vi "Auto Reziseable UI.vi"() -> ()   [LabVIEW 2010]
uses:
  <vilib>/Utility/miscctls.llb/LVPointTypeDef.ctl
  <vilib>/Utility/miscctls.llb/LVRectTypeDef.ctl
panel:
  out "Waveform Graph":i32[](graph)
  out "Front Panel Window:Window Bounds":T1
  in  "Stop Button":bool
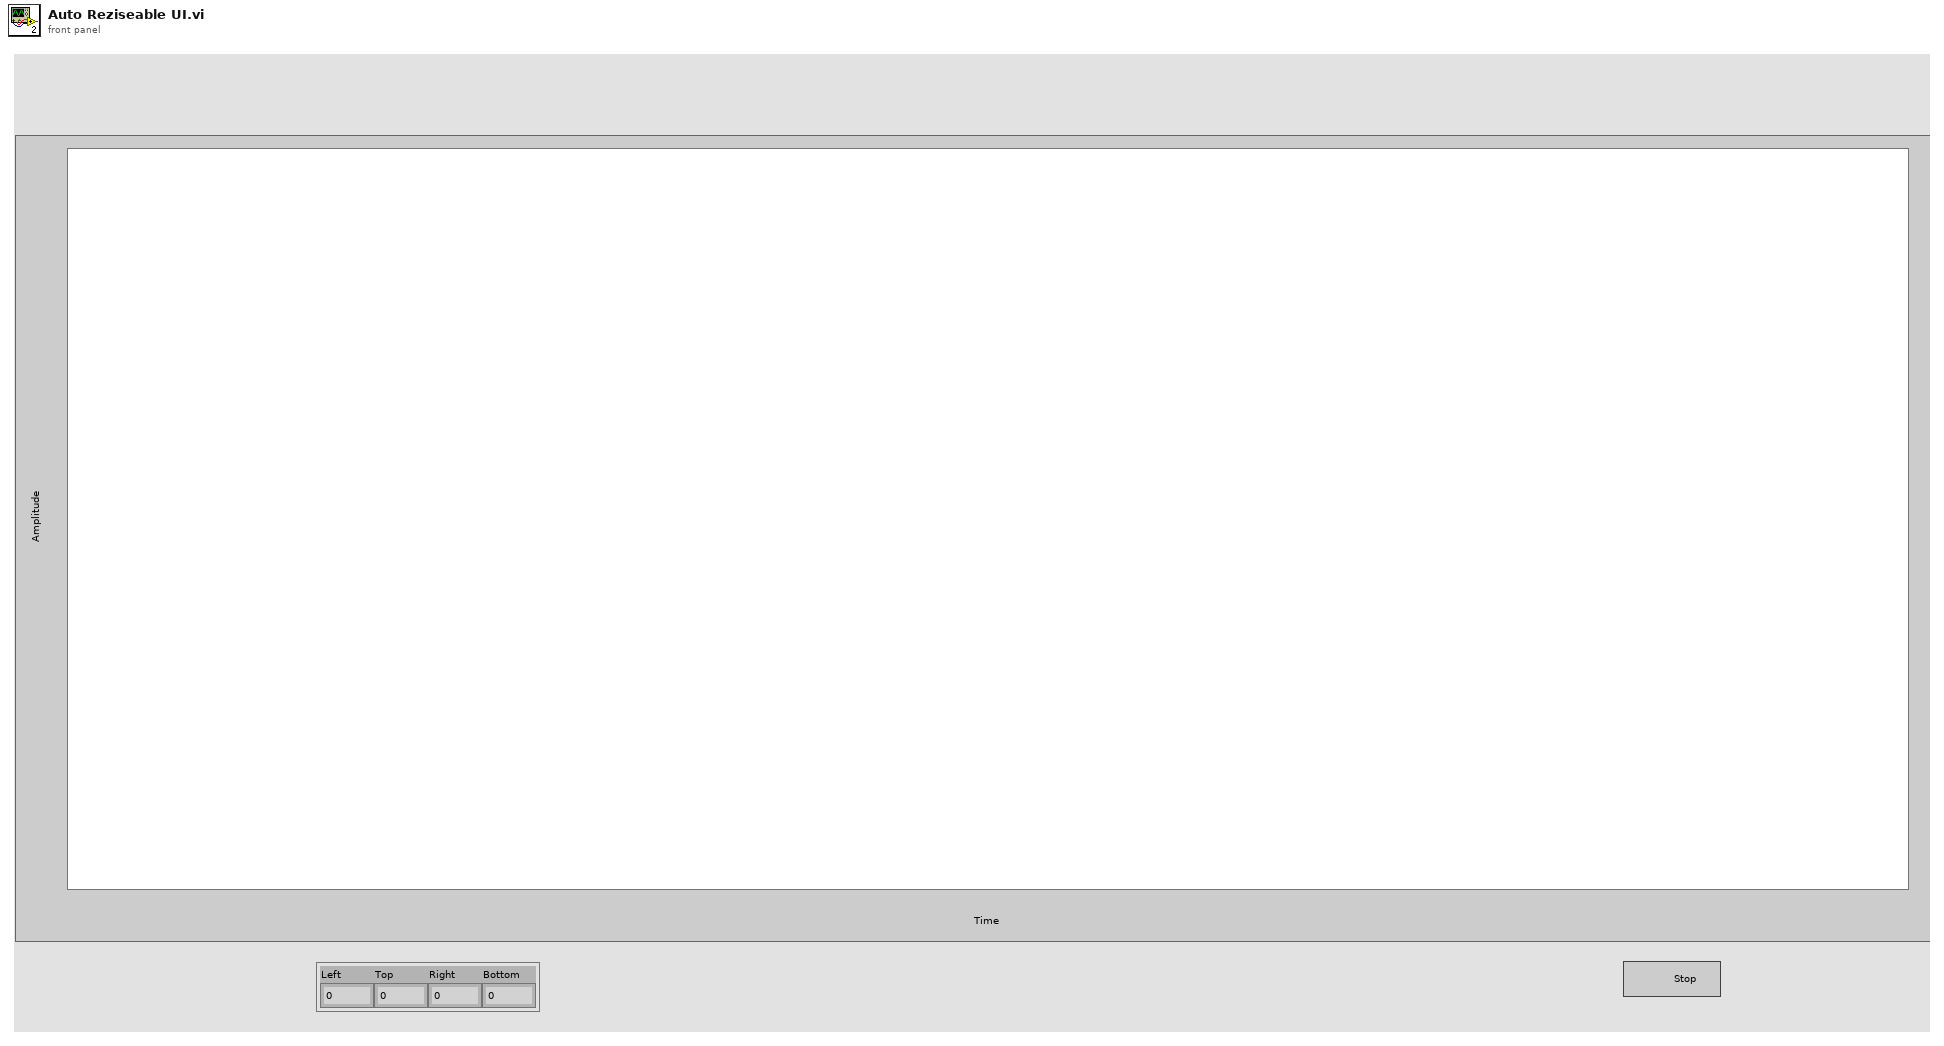
[diagram p1: front panel]
types:
  T1 = typedef "LVRectTypeDef.ctl" = cluster{"Left":i16, "Top":i16, "Right":i16, "Bottom":i16}
  T2 = typedef "LVPointTypeDef.ctl" = cluster{"Horizontal":i16, "Vertical":i16}
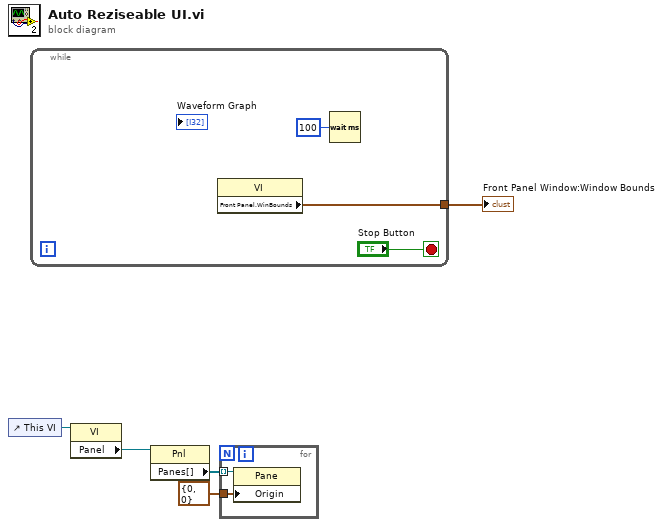
[diagram p0: block diagram]
diagram:
  n1 = control-ref of="This VI"() -> (w5:refnum<vi>)
  n2 = while {
    tunnel: [w7] -> w1
    stop <- "Stop Button" stop-if-true
    n3 = property class="VI"() -> ("Front Panel.WinBounds"=w7:T1)  [unwired: 2 in, 2 out]
    n4 = Wait (ms)(milliseconds to wait=u32 100) -> ()  [unwired: 1 out]
  }
  "Front Panel Window:Window Bounds" <- w1
  n5 = property class="VI"(reference=w5) -> ("Panel"=w2:refnum<vi>)  [unwired: 1 in, 2 out]
  n6 = property class="Pnl"(reference=w2) -> ("Panes[]"=w4:refnum<vi>[])  [unwired: 1 in, 2 out]
  n7 = for {
    tunnel: w4 -> [w10] mode=indexing
    tunnel: T2 {"Horizontal"=0, "Vertical"=0} ("Origin") -> [w9]
    n8 = property class="Pane"(reference=w10, "Origin"=w9) -> ()  [unwired: 1 in, 2 out]
  }
